vi "reset.vi"(8 "error in (no error)":errorcluster, 9 "Monochromator in":refnum<class "Monochromator.lvclass">, 11 "FaultState in":refnum<class "FaultState.lvclass">) -> (0 "error out":errorcluster, 1 "Monochromator out":refnum<class "Monochromator.lvclass">, 3 "FaultState out":refnum<class "FaultState.lvclass">)   [LabVIEW 2016, in "FaultState.lvclass"]
uses:
  FaultState.lvclass
  Monochromator/Monochromator.lvclass
  Typedefs/AckType.ctl
  Typedefs/SWStatus.ctl
  Monochromator/Monochromator.lvclass/Monochromator.ctl
panel:
  in  "Force Init":bool
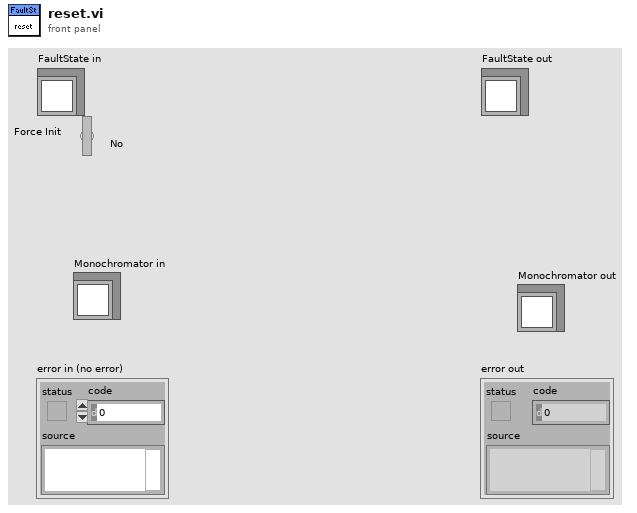
[diagram p1: front panel]
types:
  T1 = typedef "SWStatus.ctl" = enum16{"OfflineState", "ReadyState", "SettingUpState", "FaultState"}
  T2 = typedef "AckType.ctl" = enum16{"OK", "OutOfRange", "Unknown", "Busy", "Rejected"}
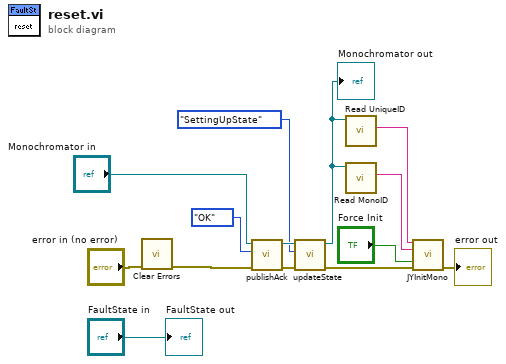
[diagram p0: block diagram]
diagram:
  n1 = call <vilib>:"Clear Errors.vi"("error in (no error)"="error in (no error)") -> ("error out"=w8:errorcluster)  [unwired: 5 in, 1 out]
  n2 = call "publishAck.vi"("error in (no error)"=w8, "Ack"=AckType."OK" ("AckType"), "Monochromator in"="Monochromator in") -> ("error out"=w5:errorcluster, "Monochromator out"=w6:refnum<class "Monochromator.lvclass">)  [unwired: 7 in]
  n3 = call "updateState.vi"("error in (no error)"=w5, "SWStatus"=SWStatus."SettingUpState", "Monochromator in"=w6) -> ("error out"=w4:errorcluster, "Monochromator out"=w2:refnum<class "Monochromator.lvclass">)  [unwired: 7 in]
  "Monochromator out" <- w2
  n4 = call "Read UniqueID.vi"("Monochromator in"=w2) -> ("UniqueID"=w12:string)  [unwired: 8 in, 2 out]
  n5 = call "Read MonoID.vi"("Monochromator in"=w2) -> ("MonoID"=w11:string)  [unwired: 8 in, 2 out]
  n6 = call "JYInitMono.vi"("Unique ID"=w12, "Mono ID"=w11, "Force Init"="Force Init", "error in (no error)"=w4) -> ("error out"=→"error out":errorcluster)  [unwired: 7 in, 4 out]
  "FaultState out" <- "FaultState in"
